vi "Get Crate Map Variables.vi"(8 "error in (no error)":errorcluster, 11 "LabVIEW Web Service Request":refnum<class "Web Request.lvclass">) -> (0 "error out":errorcluster, 3 "LabVIEW Web Service Request out":refnum<class "Web Request.lvclass">)   [LabVIEW 2018]
doc: "This VI sets all of the ESP variables for a single contact so it can be output from an ESP script."
uses:
  <vilib>/wsapi/Web Request.lvclass
  CAEN globals.vi
  subvis/i32 to dec string small.vi
  <vilib>/wsapi/class/subVIs/Set Many String ESP Variables.vi
  subvis/dbl to fr string small.vi
  <vilib>/wsapi/class/subVIs/Set Many Integer ESP Variables.vi
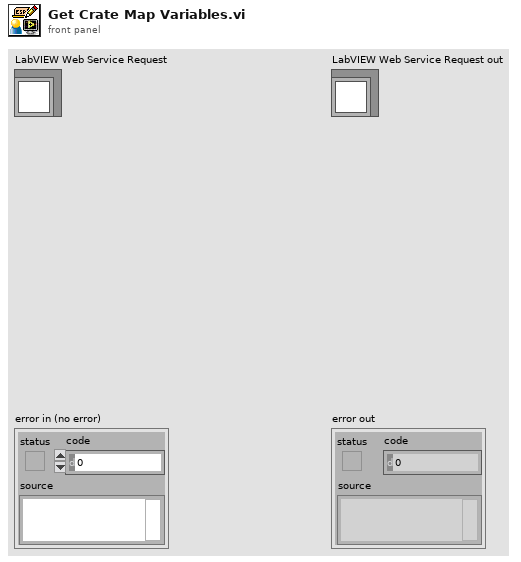
[diagram p1: front panel]
types:
  T1 = typedef "crate.ctl" = cluster{"CAENet Address":i32, "Crate Model":string, "Firmware Version":string, "Crate Map":T2[], "Total Channels":i32}
  T2 = typedef "card.ctl" = cluster{"Slot Number":i32, "Card Model":string, "Num Channels":i32, "Polarity":string, "Vmax":dbl, "Imax":dbl, "Revision":string}
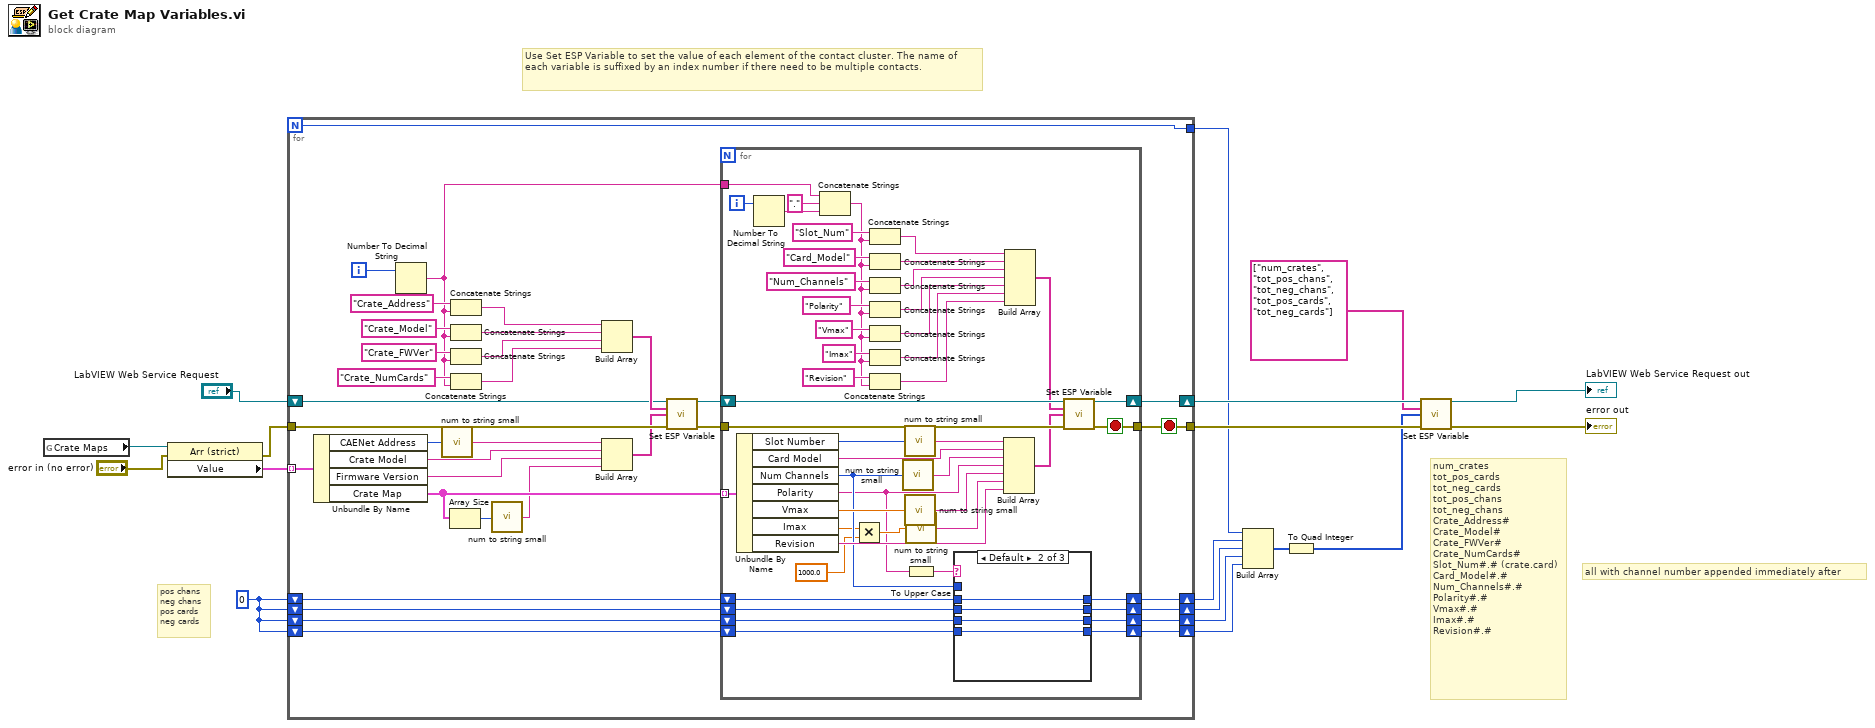
[diagram p0: block diagram]
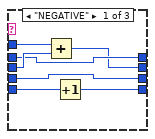
[diagram p2: hidden frame]
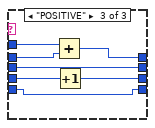
[diagram p3: hidden frame]
diagram:
  w12 = 0 ("CAENet Address")
  # "pos chans\nneg chans\npos cards\nneg cards"
  # "all with channel number appended immediately after"
  # "num_crates\ntot_pos_cards\ntot_neg_cards\ntot_pos_chans\ntot_neg_chans\nCrate_Address#\nCrate_Model#\nCrate_FWVer#\nCrate_NumCards#\nSlot_Num#.# (crate.card)\nCard_Model#.#\nNum_Channels#.#\nPolarity#.#\nVmax#.#\nImax#.#\nRevision#.#"
  # "Use Set ESP Variable to set the value of each element of the contact cluster. The name of each variable is suffixed by an index number if there need to be multiple contacts."
  n1 = global read "CAEN globals.vi" "Crate Maps"() -> (w4:refnum<vi>)
  n2 = property class="Arr (strict)"(reference=w4, error in="error in (no error)") -> (error out=w1:errorcluster, "Value"=w3:T1[])  [unwired: 1 out]
  n3 = for {
    N -> [w40]
    tunnel: w3 -> [w42] mode=indexing
    tunnel: w1 -> [w53]
    tunnel: [w33] -> w17
    tunnel: [w40] -> w7
    shift-right: [w35] -> w16
    shift-left: "LabVIEW Web Service Request" -> [w45]
    shift-right: [w22] -> w11
    shift-left: w12 -> [w26]
    shift-right: [w21] -> w10
    shift-left: w12 -> [w25]
    shift-right: [w20] -> w9
    shift-left: w12 -> [w24]
    shift-right: [w19] -> w8
    shift-left: w12 -> [w23]
    i -> [w41]
    stop <- w33 stop-if-true
    n4 = Unbundle By Name(w42) -> ("CAENet Address"=w39:i32, "Crate Model"=w38:string, "Firmware Version"=w37:string, "Crate Map"=w32:T2[])
    n5 = Number To Decimal String(number=w41) -> (decimal integer string=w28:string)  [unwired: 1 in]
    n6 = call-poly "num to string small.vi"("number"=w39) -> ("String"=w44:string)  [unwired: 14 in]
    n7 = Array Size(array=w32) -> (size(s)=w31:i32)
    n8 = Concatenate Strings("Crate_Address" ("string"), w28) -> (w43:string)
    n9 = Concatenate Strings("Crate_Model" ("string"), w28) -> (w49:string)
    n10 = Concatenate Strings("Crate_FWVer" ("string"), w28) -> (w48:string)
    n11 = Concatenate Strings("Crate_NumCards" ("string"), w28) -> (w27:string)
    n12 = call-poly "num to string small.vi"("number"=w31) -> ("String"=w30:string)  [unwired: 14 in]
    n13 = Build Array(w43, w49, w48, w27) -> (w47:string[])
    n14 = Build Array(w44, w38, w37, w30) -> (w46:string[])
    n15 = call-poly <vilib>:"Set ESP Variable.vi"("LabVIEW Web Service Request"=w45, "keys"=w47, "values"=w46, "error in (no error)"=w53) -> ("LabVIEW Web Service Request out"=w36:refnum<class "Web Request.lvclass">, "error out"=w34:errorcluster)  [unwired: 10 in]
    n16 = for {
      shift-right: [w100] -> w35
      shift-left: w36 -> [w101]
      tunnel: w34 -> [w99]
      tunnel: [w98] -> w33
      tunnel: w32 -> [w82] mode=indexing
      tunnel: w28 -> [w71]
      shift-right: [w62] -> w22
      shift-left: w26 -> [w66]
      shift-right: [w61] -> w21
      shift-left: w25 -> [w65]
      shift-right: [w60] -> w20
      shift-left: w24 -> [w64]
      shift-right: [w59] -> w19
      shift-left: w23 -> [w63]
      i -> [w72]
      stop <- w98 stop-if-true
      n17 = Unbundle By Name(w82) -> ("Slot Number"=w80:i32, "Card Model"=w78:string, "Num Channels"=w67:i32, "Polarity"=w55:string, "Vmax"=w81:dbl, "Imax"=w58:dbl, "Revision"=w74:string)
      n18 = Number To Decimal String(number=w72) -> (decimal integer string=w70:string)  [unwired: 1 in]
      n19 = Concatenate Strings(w71, "." ("string"), w70) -> (w68:string)
      n20 = Multiply(x=w58, y=1000.0) -> (x*y=w57:dbl)
      n21 = Concatenate Strings("Slot_Num" ("string"), w68) -> (w84:string)
      n22 = Concatenate Strings("Card_Model" ("string"), w68) -> (w90:string)
      n23 = Concatenate Strings("Num_Channels" ("string"), w68) -> (w89:string)
      n24 = Concatenate Strings("Polarity" ("string"), w68) -> (w88:string)
      n25 = Concatenate Strings("Vmax" ("string"), w68) -> (w87:string)
      n26 = Concatenate Strings("Imax" ("string"), w68) -> (w86:string)
      n27 = Concatenate Strings("Revision" ("string"), w68) -> (w85:string)
      n28 = call-poly "num to string small.vi"("number"=w67) -> ("String"=w77:string)  [unwired: 14 in]
      n29 = call-poly "num to string small.vi"("number"=w80) -> ("String"=w79:string)  [unwired: 14 in]
      n30 = call-poly "num to string small.vi"("number"=w81) -> ("String"=w76:string)  [unwired: 14 in]
      n31 = call-poly "num to string small.vi"("number"=w57) -> ("String"=w75:string)  [unwired: 14 in]
      n32 = To Upper Case(1:w55) -> (0:w54:string)
      n33 = case shown="Default" w54 {
        tunnel: w67 -> [w108 _ w119]
        tunnel: w66 -> [w106 w112 w118]
        tunnel: w65 -> [w107 w111 w116]
        tunnel: w64 -> [w102 w110 w115]
        tunnel: w63 -> [w104 w109 w113]
        tunnel: [w106 w112 w117] -> w62
        tunnel: [w105 w111 w116] -> w61
        tunnel: [w102 w110 w114] -> w60
        tunnel: [w103 w109 w113] -> w59
        frame "NEGATIVE" {
          n34 = Add(x=w108, y=w107) -> (x+y=w105:i32)
          n35 = Increment(x=w104) -> (x+1=w103:i32)
        }
        frame Default {
        }
        frame "POSITIVE" {
          n36 = Add(x=w119, y=w118) -> (x+y=w117:i32)
          n37 = Increment(x=w115) -> (x+1=w114:i32)
        }
      }
      n38 = Build Array(w79, w78, w77, w55, w76, w75, w74) -> (w73:string[])
      n39 = Build Array(w84, w90, w89, w88, w87, w86, w85) -> (w83:string[])
      n40 = call-poly <vilib>:"Set ESP Variable.vi"("LabVIEW Web Service Request"=w101, "keys"=w83, "values"=w73, "error in (no error)"=w99) -> ("LabVIEW Web Service Request out"=w100:refnum<class "Web Request.lvclass">, "error out"=w98:errorcluster)  [unwired: 10 in]
    }
  }
  n41 = Build Array(w7, w11, w10, w9, w8) -> (w6:i32[])
  n42 = To Quad Integer(1:w6) -> (0:w15:i64[])
  n43 = call-poly <vilib>:"Set ESP Variable.vi"("LabVIEW Web Service Request"=w16, "keys"=string[] ["num_crates", "tot_pos_chans", "tot_neg_chans", "tot_pos_cards", "tot_neg_cards"] ("appended array"), "values"=w15, "error in (no error)"=w17) -> ("LabVIEW Web Service Request out"=→"LabVIEW Web Service Request out":refnum<class "Web Request.lvclass">, "error out"=→"error out":errorcluster)  [unwired: 10 in]
